vi "Pachube Datapoints PUT LaunchPad.vi"(10 "Pachube datastream ID":string="0", 11 "Value":dbl) -> (2 "Error code":i32, 3 "Error":bool)   [LabVIEW 2010]
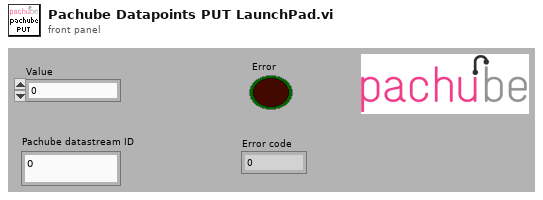
[diagram p1: front panel]
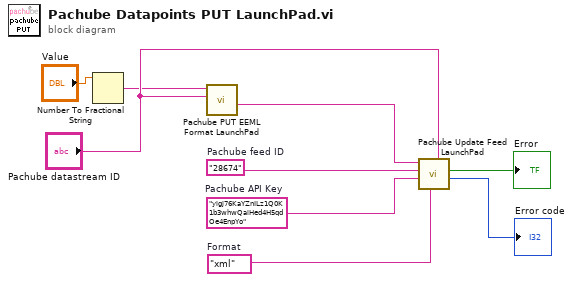
[diagram p0: block diagram]
diagram:
  w9 = "28674"  # Pachube feed ID
  w8 = "yigj76KaYZnILz1Q0K1b3whwQaiHed4H5qdOe4EnpYo"  # Pachube API Key
  w7 = "xml"  # Format
  n1 = Number To Fractional String(number="Value") -> (F-format string=w2:string)  [unwired: 3 in]
  n2 = call "Pachube PUT EEML Format LaunchPad.vi"("Pachube datastream ID"="Pachube datastream ID", "Value"=w2) -> ("Data"=w6:string)  [unwired: 9 in]
  n3 = call "Pachube Update Feed LaunchPad.vi"("Pachube datastream ID"="Pachube datastream ID", "Format"=w7, "Pachube API Key"=w8, "Pachube feed ID"=w9, "Data"=w6) -> ("Error code"=→"Error code":i32, "Error"=→"Error":bool)  [unwired: 4 in, 1 out]
